vi "ASC-OvershootTest.vi"() -> ()   [LabVIEW 2009]
uses:
  <vilib>/Utility/error.llb/DialogType.ctl
  Time_globals.vi
panel:
  out "log fO2 rel. IW/IM":dbl
  out "Flush":bool
  out "Progress":string
  in  "Fugacity table":dbl[](array[numeric])
  in  "Temperature table":dbl[](array[numeric])
  out "Fugacity":cluster{"Array":dbl[], "Array 2":dbl[]}[](graph)=[{"Array"=[17.44743958824043, 17.44743958824043], "Array 2"=[-15.0, -90.0]}, {"Array"=[14.85552997103172, 14.85552997103172], "Array 2"=[-15.0, -90.0]}, {"Array"=[12.93410075664489, 12.93410075664489], "Array 2"=[-15.0, -90.0]}, {"Array"=[11.45278589016778, 11.45278589016778], "Array 2"=[-15.0, -90.0]}, {"Array"=[10.27590813338129, 10.27590813338129], "Array 2"=[-15.0, -90.0]}, {"Array"=[9.318361831989936, 9.318361831989936], "Array 2"=[-15.0, -90.0]}, {"Array"=[21.13, 21.13], "Array 2"=[-15.0, -90.0]}, {"Array"=[26.8, 26.8], "Array 2"=[-15.0, -90.0]}, {"Array"=[33.65, 33.65], "Array 2"=[-15.0, -90.0]}, {"Array"=[9.0, 11.83374083129584, 33.65, 33.65], "Array 2"=[-17.9235, -25.63552567237164, -89.48, -89.48]}, {"Array"=[], "Array 2"=[]}] caption="XY Graph"
  out "Datafile blob":string="8/29/2014\t3:28 PM\r\n\r\n0*C\r\nH2-CO2\r\nIW/IM+0\r\n\r\nTime\tSet_point\tLoad_end\tSample\tFan_end\tFan\tField\t%CO2\r\n"
  out "Start":bool
  out "Cool":bool
  out "Stable":bool
  in  "stop":bool
  out "Current SP":dbl=50.0
  out "Array":dbl[](array[numeric])
  out "refnum out":refnum<file>
  out "Fan on":bool
  in  "FAN":bool caption="Fan"
  in  "error in":errorcluster
  out "Set Point (*C)":u32
  out "Elapsed Time":dbl format="%#.0f"
  out "fan end":u32
  out "load end":u32
  out "sample":u32
  out "Watlow Chart":T1(graph)={"Number"=133, "Number"=270, "Number"=56}
  # "Temperature"
  # "Current\nTemperature"
  # "800"
  # "700"
  # "600"
  # "500"
  # "400"
  # "300"
  # "200"
  # "100"
  # "20"
  # "Temperature (*C)"
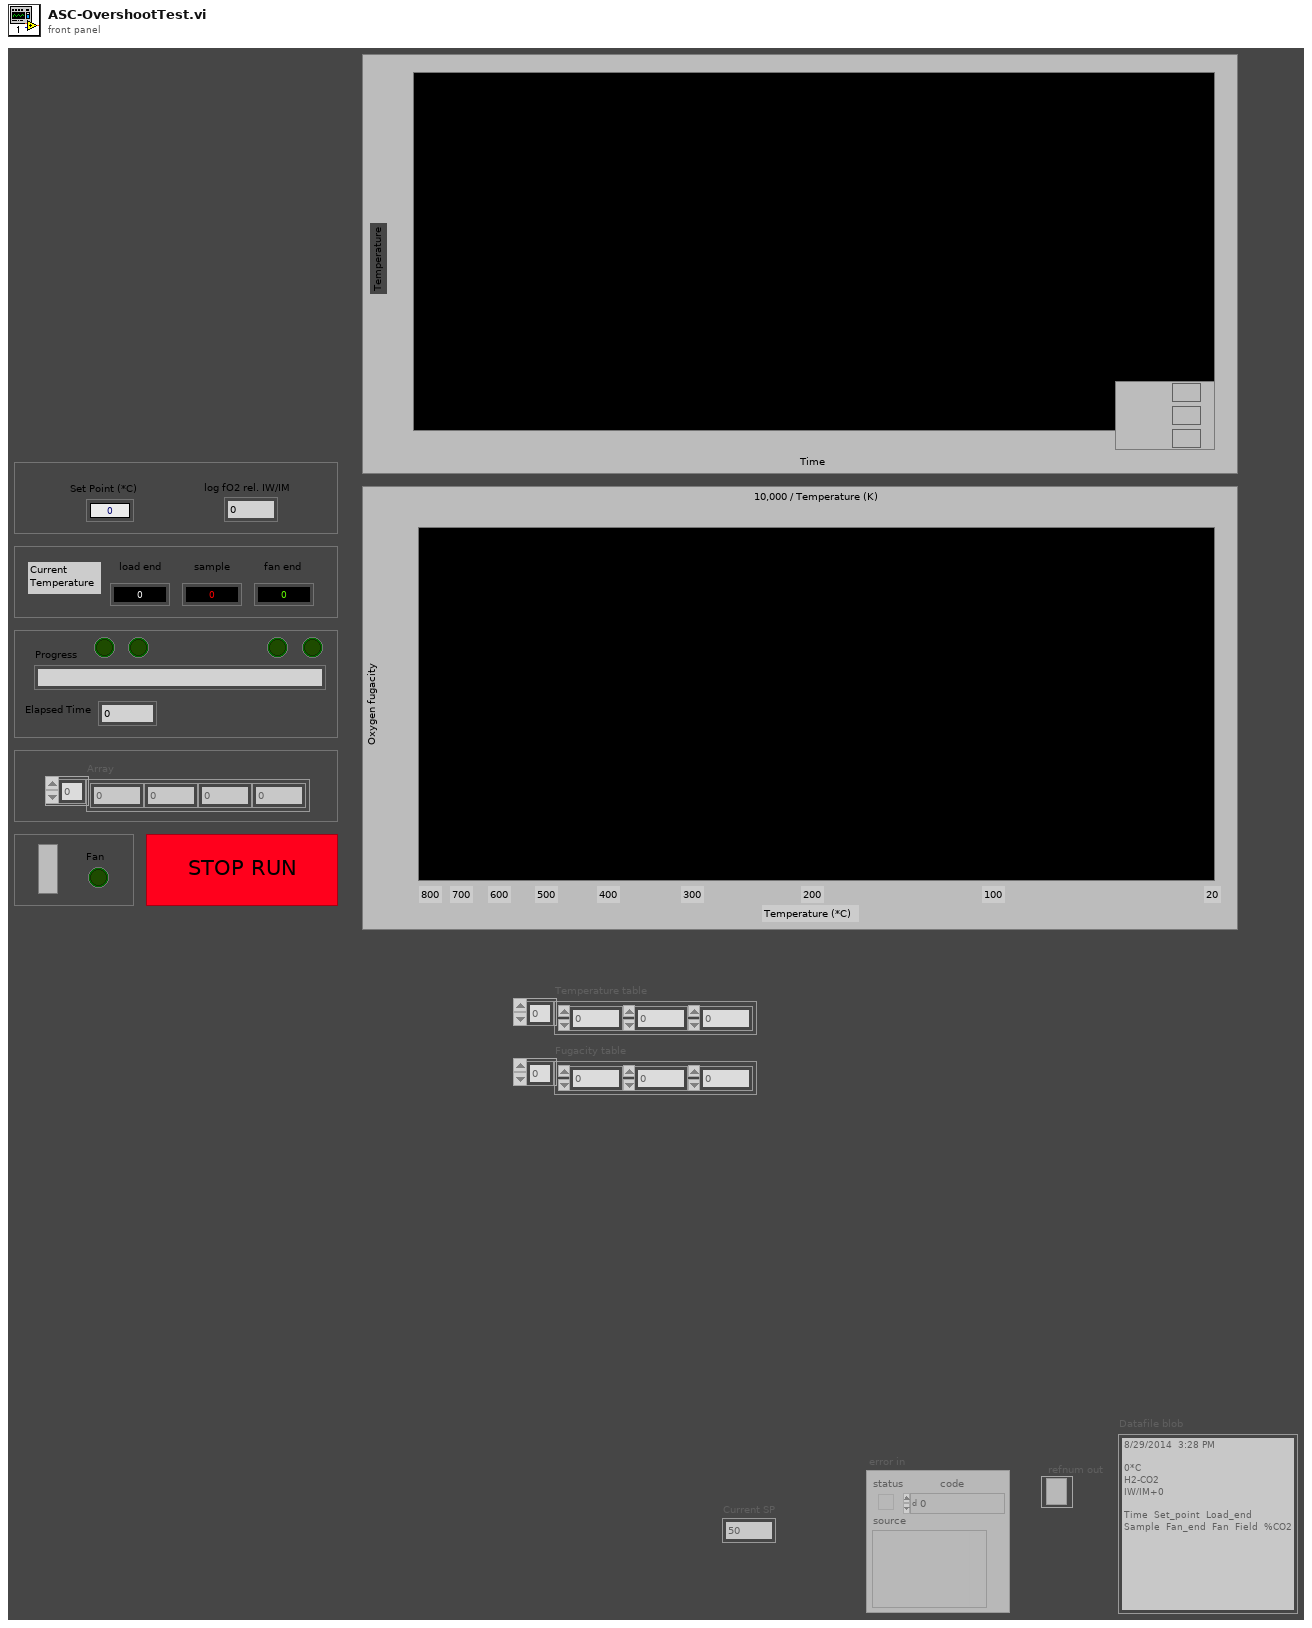
[diagram p1: front panel]
types:
  T1 = cluster{"Number":u32, "Number":u32, "Number":u32}
  T2 = cluster{"Number":u32, "Number":u32, "Number":u32}[]
  T3 = cluster{"Flow Controllers":refnum<visa-resource-name>, "Oven Fan":refnum<visa-resource-name>, "Oven Watlows":refnum<visa-resource-name>, "Field Power Supply":refnum<visa-resource-name>}
  T4 = typedef "DialogType.ctl" = u16
  T5 = cluster{"Oven Watlows":refnum<visa-resource-name>, "Field Power Supply":refnum<visa-resource-name>, "Oven Fan":refnum<visa-resource-name>, "Flow Controllers":refnum<visa-resource-name>}
  T6 = cluster{"Set Point (*C)":u32, "Number":u32, "refnum out":refnum<file>}
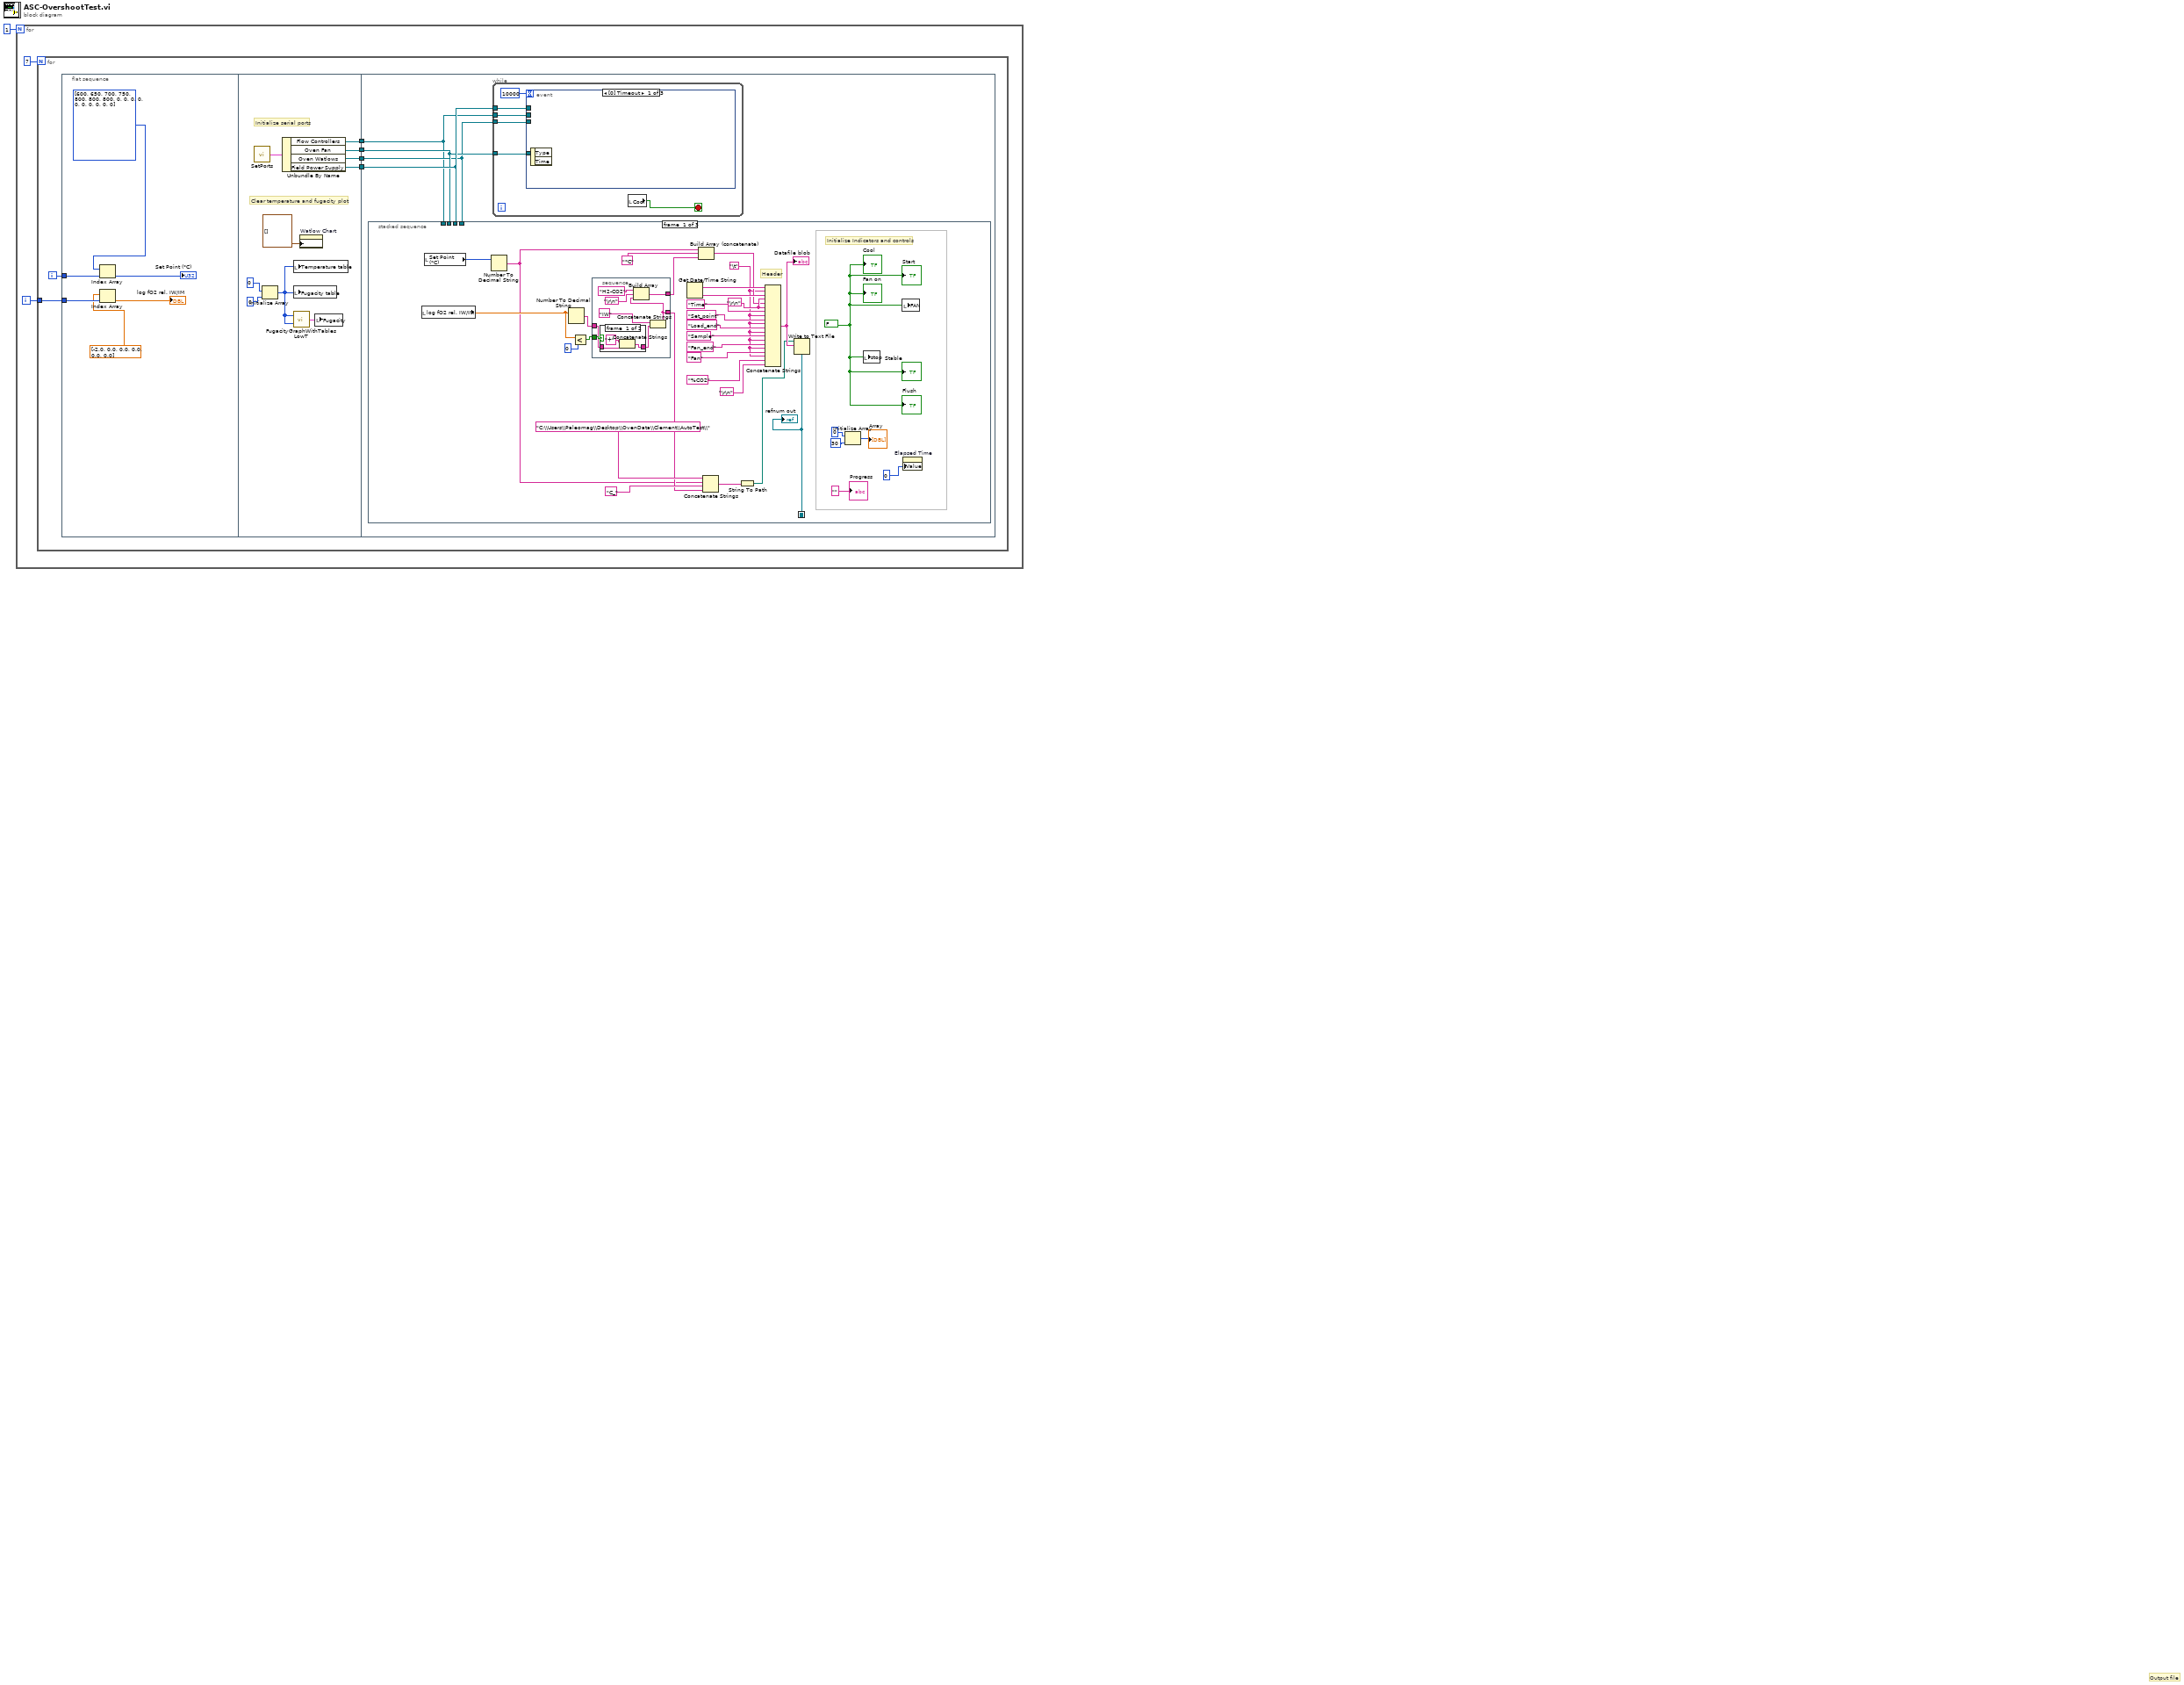
[diagram p0: block diagram]
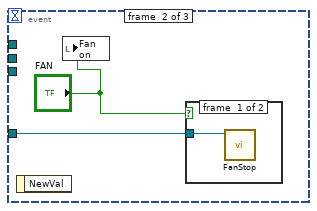
[diagram p2: hidden frame]
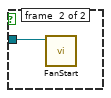
[diagram p3: hidden frame]
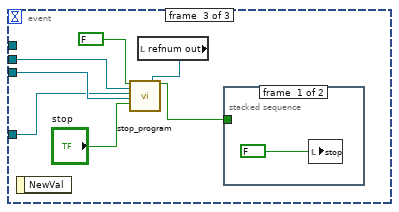
[diagram p4: hidden frame]
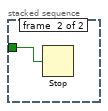
[diagram p5: hidden frame]
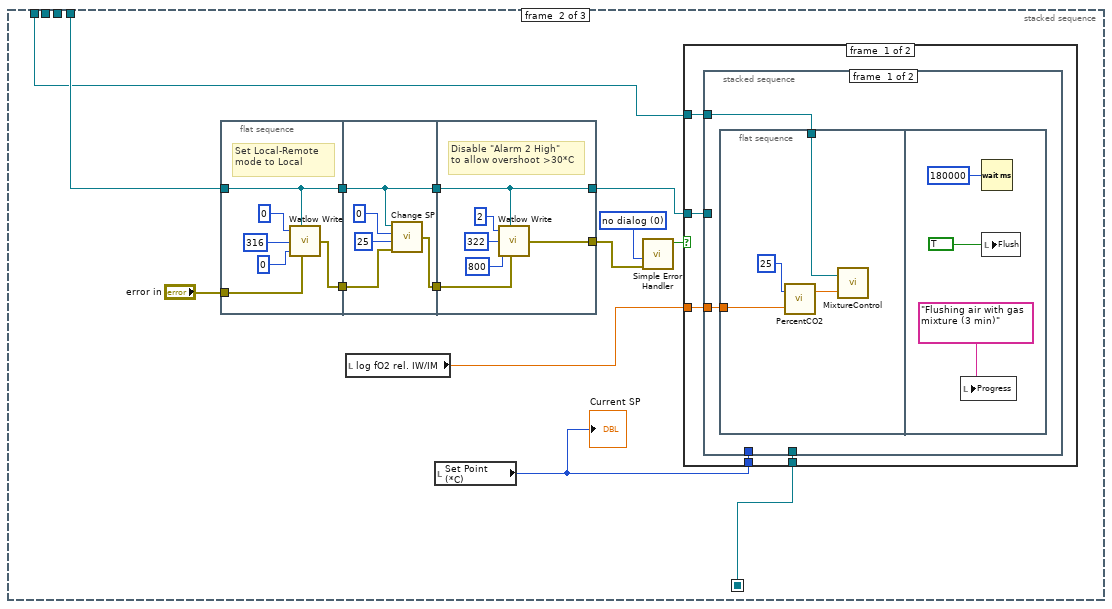
[diagram p7: hidden frame]
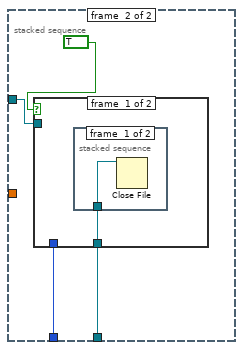
[diagram p8: hidden frame]
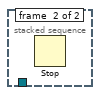
[diagram p9: hidden frame]
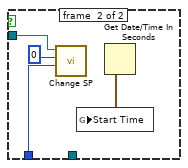
[diagram p10: hidden frame]
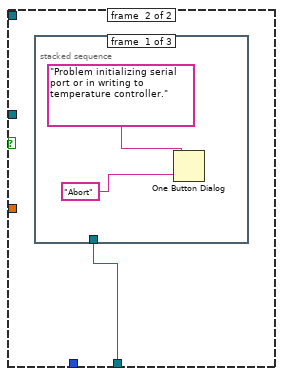
[diagram p11: hidden frame]
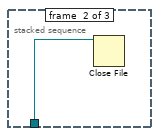
[diagram p12: hidden frame]
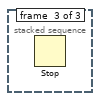
[diagram p13: hidden frame]
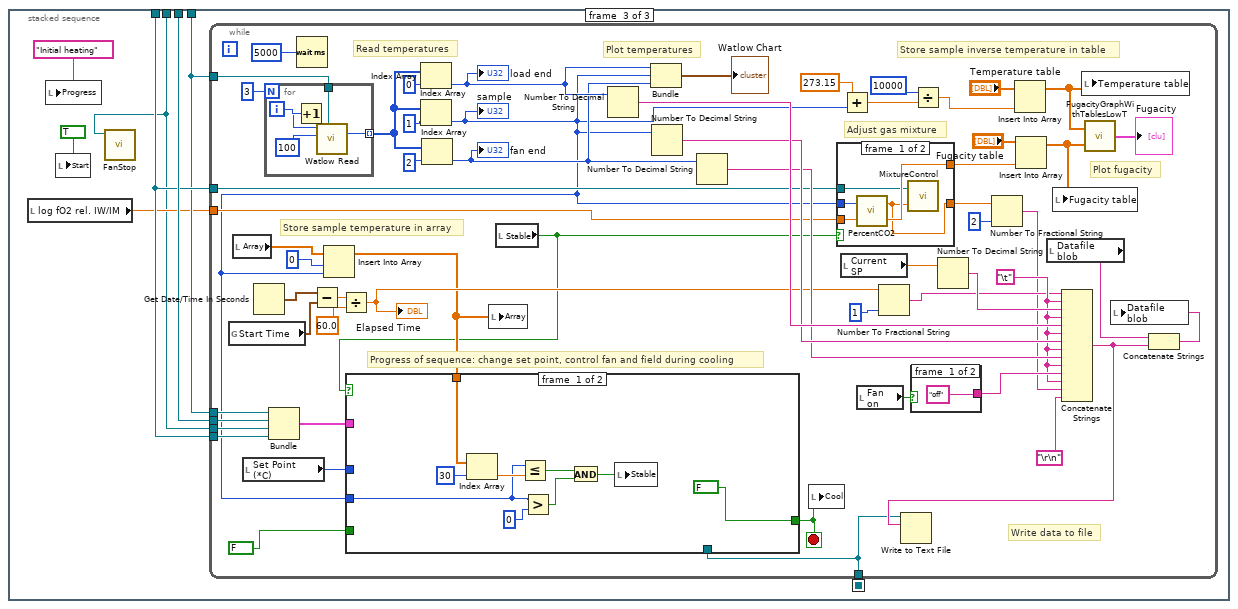
[diagram p14: hidden frame]
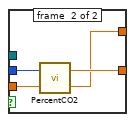
[diagram p15: hidden frame]
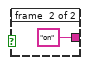
[diagram p16: hidden frame]
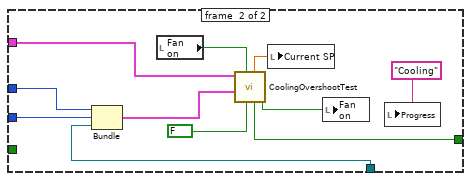
[diagram p17: hidden frame]
diagram:
  # "Output file"
  n1 = for {
    N: 1 -> [_]
    i -> [w3]
    n2 = for {
      N: 7 -> [_]
      tunnel: w3 -> [w4]
      i -> [w5]
      n3 = flat-sequence {
        tunnel: w5 -> [w15]
        tunnel: w4 -> [w14]
        tunnel: [w24] -> w9
        tunnel: [w23] -> w8
        tunnel: [w22] -> w7
        tunnel: [w19] -> w6
        tunnel: w9 -> [w29]
        tunnel: w8 -> [w28]
        tunnel: w7 -> [w27]
        tunnel: w6 -> [w26]
        frame #0 {
          n4 = Index Array(array=i32[] [600, 650, 700, 750, 800, 800, 800, 0, 0, 0, 0, 0, 0, 0, 0, 0, 0], index=w15) -> (element=→"Set Point (*C)":i32)
          n5 = Index Array(array=dbl[] [-2.0, 0.0, 0.0, 0.0, 0.0, 0.0], index=w14) -> (element=→"log fO2 rel. IW/IM":dbl)
        }
        frame #1 {
          # "Clear temperature and fugacity plot"
          # "Initialize serial ports"
          n6 = call "SetPorts.vi"() -> ("Ports"=w25:T3)  [unwired: 1 in]
          n7 = Initialize Array(0, 0) -> (w18:i32[])
          n8 = Unbundle By Name(w25) -> ("Flow Controllers"=w19:refnum<visa-resource-name>, "Oven Fan"=w23:refnum<visa-resource-name>, "Oven Watlows"=w22:refnum<visa-resource-name>, "Field Power Supply"=w24:refnum<visa-resource-name>)
          n9 = local write "Temperature table"(w18) -> ()
          n10 = local write "Fugacity table"(w18) -> ()
          n11 = call "FugacityGraphWithTablesLowT.vi"("Fugacity table"=w18, "Temperature table"=w18) -> ("Array"=w17:cluster{"Array":dbl[], "Array 2":dbl[]}[])
          n12 = property on="Watlow Chart" class="WaveformChart (strict)"("History Data"=T2 []) -> ()  [unwired: 2 in, 2 out]
          n13 = local write "Fugacity"(w17) -> ()
        }
        frame #2 {
          n14 = stacked-sequence {
            seq-local: [w58 _ _] -> [_ w98 w161]
            tunnel: w27 -> [_ w105 w156]
            tunnel: w28 -> [_ _ w154]
            tunnel: w29 -> [_ _ w159]
            tunnel: w26 -> [_ w97 w157]
            frame #0 {
              w74 = "\r\n" ("End of Line Constant")
              w61 = "\t" ("Tab Constant")
              w57 = FALSE
              # "Header"
              # "Initialize Indicators and controls"
              n15 = local read "log fO2 rel. IW/IM"() -> (w51:dbl)
              n16 = local read "Set Point (*C)"() -> (w50:u32)
              n17 = Number To Decimal String(number=w50) -> (decimal integer string=w49:string)  [unwired: 1 out]
              n18 = Number To Decimal String(number=w51) -> (decimal integer string=w65:string)  [unwired: 1 out]
              n19 = Less?(x=w51, y=0) -> (x < y?=w63:bool)
              n20 = stacked-sequence {
                tunnel: [w89] -> w70
                tunnel: w65 -> [w85]
                tunnel: w63 -> [w86]
                tunnel: [w83] -> w52
                frame #0 {
                  n21 = case shown="True" w86 {
                    tunnel: w85 -> [w92 w94]
                    tunnel: [w91 w94] -> w84
                    frame #0 {
                      n22 = Concatenate Strings("+", w92) -> (w91:string)
                    }
                    frame #1 {
                    }
                  }
                  n23 = Concatenate Strings("IW", w84) -> (w83:string)
                  n24 = Build Array("H2-CO2", "\r\n" ("End of Line Constant"), w83) -> (w89:string[])
                }
              }
              n25 = Get Date/Time String() -> (date string=w76:string, time string=w75:string)  [unwired: 3 out]
              n26 = Build Array (concatenate)(w49, "*C", w70) -> (w69:string[])
              n27 = Concatenate Strings("C:\\Users\\Paleomag\\Desktop\\OvenData\\Clement\\AutoTest\\", w49, "C_", w52) -> (w56:string)
              n28 = String To Path(string=w56) -> (path=w54:path)
              n29 = Concatenate Strings(w76, w61, w75, w74, w69, w74, "Time", w61, "Set_point", w61, "Load_end", w61, "Sample", w61, "Fan_end", w61, "Fan", w61, "%CO2", "\r\n") -> (w62:string)
              "Datafile blob" <- w62
              n30 = Write to Text File(file (use dialog)=w54, text=w62) -> (refnum out=w58:refnum<file>)  [unwired: 1 in, 3 out]
              "refnum out" <- w58
              n31 = Initialize Array(0, 30) -> (→"Array":i32[])
              n32 = local write "stop"(w57) -> ()
              n33 = local write "FAN"(w57) -> ()
              n34 = property on="Elapsed Time" class="DigNum (strict)"("Value"=0) -> ()  [unwired: 2 in, 2 out]
              "Fan on" <- w57
              "Cool" <- w57
              "Stable" <- w57
              "Start" <- w57
              "Flush" <- w57
              "Progress" <- ""
            }
            frame #1 {
              w108 = T4 0 items=["no dialog", "OK message", "continue or stop message", "OK message + warnings", "continue/stop + warnings"] ("type of dialog (OK msg:1)")
              n35 = flat-sequence {
                tunnel: w105 -> [w111]
                tunnel: [w111] -> w103
                tunnel: "error in" -> [w110]
                tunnel: [w109] -> w101
                tunnel: w103 -> [w119]
                tunnel: [w119] -> w102
                tunnel: w101 -> [w116]
                tunnel: [w115] -> w100
                tunnel: w102 -> [w120]
                tunnel: w100 -> [w125]
                tunnel: [w121] -> w99
                tunnel: [w120] -> w104
                frame #0 {
                  # "Set Local-Remote\nmode to Local"
                  n36 = call "Watlow Write.vi"("Adress"=0, "VISA resource name"=w111, "Register"=316, "Parameter"=0, "error in (no error)"=w110) -> ("error out"=w109:errorcluster)
                }
                frame #1 {
                  n37 = call "Change SP.vi"("error in"=w116, "Set Point"=25, "Adress"=0, "VISA resource name"=w119) -> ("error out"=w115:errorcluster)
                }
                frame #2 {
                  # "Disable \"Alarm 2 High\"\nto allow overshoot >30*C"
                  n38 = call "Watlow Write.vi"("Adress"=2, "VISA resource name"=w120, "Register"=322, "Parameter"=800, "error in (no error)"=w125) -> ("error out"=w121:errorcluster)
                }
              }
              n39 = local read "log fO2 rel. IW/IM"() -> (w96:dbl)
              n40 = local read "Set Point (*C)"() -> (w95:u32)
              "Current SP" <- w95
              n41 = call <vilib>:"Simple Error Handler.vi"("type of dialog (OK msg:1)"=w108, "error in (no error)"=w99) -> ("error?"=w107:bool)  [unwired: 7 out]
              n42 = case shown="False" w107 {
                tunnel: w98 -> [w130 w150]
                tunnel: w104 -> [w129 _]
                tunnel: w95 -> [w128 _]
                tunnel: w96 -> [w127 _]
                tunnel: w97 -> [w126 _]
                frame #0 {
                  n43 = stacked-sequence {
                    tunnel: w130 -> [_ w143]
                    tunnel: w129 -> [_ w142]
                    tunnel: w128 -> [_ w141]
                    tunnel: w127 -> [w131 _]
                    tunnel: w126 -> [w132 _]
                    frame #0 {
                      n44 = flat-sequence {
                        tunnel: w132 -> [w136]
                        tunnel: w131 -> [w133]
                        frame #0 {
                          n45 = call "PercentCO2.vi"("log fO2 rel. IW/IM"=w133, "Temperature"=25) -> ("%CO2"=w135:dbl)  [unwired: 1 out]
                          n46 = call "MixtureControl.vi"("%CO2"=w135, "VISA resource name"=w136) -> ()  [unwired: 1 in]
                        }
                        frame #1 {
                          n47 = local write "Progress"("Flushing air with gas mixture (3 min)") -> ()
                          n48 = Wait (ms)(milliseconds to wait=180000) -> ()  [unwired: 1 out]
                          n49 = local write "Flush"(TRUE) -> ()
                        }
                      }
                    }
                    frame #1 {
                      n50 = case shown="True" TRUE {
                        tunnel: w143 -> [w144 _]
                        tunnel: w142 -> [_ w148]
                        tunnel: w141 -> [_ w147]
                        frame #0 {
                          n51 = stacked-sequence {
                            tunnel: w144 -> [w145 _]
                            frame #0 {
                              n52 = Close File(refnum=w145) -> ()  [unwired: 1 in, 2 out]
                            }
                            frame #1 {
                              n53 = Stop() -> ()  [unwired: 1 out]
                            }
                          }
                        }
                        frame #1 {
                          n54 = call "Change SP.vi"("Set Point"=w147, "Adress"=0, "VISA resource name"=w148) -> ()  [unwired: 1 in, 1 out]
                          n55 = Get Date/Time In Seconds() -> (seconds since 1Jan1904=w149:timestamp)
                          n56 = global write "Time_globals.vi" "Start Time"(w149) -> ()
                        }
                      }
                    }
                  }
                }
                frame #1 {
                  n57 = stacked-sequence {
                    tunnel: w150 -> [_ w153 _]
                    frame #0 {
                      n58 = One Button Dialog(message="Problem initializing serial port or in writing to temperature controller.", button name ("OK")="Abort") -> ()  [unwired: 1 out]
                    }
                    frame #1 {
                      n59 = Close File(refnum=w153) -> ()  [unwired: 1 in, 2 out]
                    }
                    frame #2 {
                      n60 = Stop() -> ()  [unwired: 1 out]
                    }
                  }
                }
              }
            }
            frame #2 {
              n61 = local read "log fO2 rel. IW/IM"() -> (w155:dbl)
              n62 = local write "Progress"("Initial heating") -> ()
              n63 = local write "Start"(TRUE) -> ()
              n64 = call "FanStop.vi"("VISA resource name"=w154) -> ()  [unwired: 11 in]
              n65 = while {
                tunnel: w161 -> [w198]
                tunnel: w156 -> [w181]
                tunnel: w159 -> [w174]
                tunnel: w154 -> [w173]
                tunnel: w155 -> [w192]
                tunnel: w157 -> [w172]
                tunnel: w157 -> [w176]
                tunnel: w156 -> [w175]
                stop <- w180 stop-if-true
                w182 = "\t"
                # "Store sample temperature in array"
                # "Write data to file"
                # "Progress of sequence: change set point, control fan and field during cooling"
                # "Adjust gas mixture"
                # "Plot fugacity"
                # "Store sample inverse temperature in table"
                # "Plot temperatures"
                # "Read temperatures"
                n66 = global read "Time_globals.vi" "Start Time"() -> (w206:timestamp)
                n67 = local read "Array"() -> (w179:dbl[])
                n68 = local read "Set Point (*C)"() -> (w164:u32)
                n69 = Get Date/Time In Seconds() -> (seconds since 1Jan1904=w205:timestamp)
                n70 = for {
                  N: 3 -> [_]
                  tunnel: [w253] -> w214 mode=indexing
                  tunnel: w181 -> [w252]
                  i -> [w255]
                  n71 = Increment(x=w255) -> (x+1=w254:i32)
                  n72 = call "Watlow Read.vi"("Adress"=w254, "Register"=u8 100 ("ST-H"), "VISA resource name"=w252) -> ("Number"=w253:u32)  [unwired: 1 in, 2 out]
                }
                n73 = Bundle("Oven Watlows"=w175, "Field Power Supply"=w174, "Oven Fan"=w173, "Flow Controllers"=w172) -> (w171:T5)  [unwired: 1 in]
                n74 = Wait (ms)(milliseconds to wait=u32 5000) -> ()  [unwired: 1 out]
                n75 = Subtract(x=w205, y=w206) -> (x-y=w207:dbl)
                n76 = Divide(x=w207, y=60.0) -> (x/y=w204:dbl)
                "Elapsed Time" <- w204
                n77 = Index Array(array=w214, index=0) -> (element=w210:u32)
                "load end" <- w210
                n78 = Index Array(array=w214, index=1) -> (element=w167:u32)
                "sample" <- w167
                n79 = Insert Into Array(array=w179, index=0, new element=w167) -> (w163:dbl[])
                n80 = Index Array(array=w214, index=2) -> (element=w209:u32)
                "fan end" <- w209
                n81 = local write "Array"(w163) -> ()
                n82 = local read "Stable"() -> (w162:bool)
                n83 = case shown="False" w162 {
                  tunnel: w198 -> [_ w243]
                  tunnel: [FALSE w247] -> w180
                  tunnel: w164 -> [_ w249]
                  tunnel: w167 -> [w235 w248]
                  tunnel: FALSE -> [_ _]
                  tunnel: w163 -> [w237 _]
                  tunnel: w171 -> [_ w242]
                  frame #0 {
                    n84 = Index Array(array=w237, index=30) -> (element=w238:dbl)
                    n85 = Less Or Equal?(x=w235, y=w238) -> (x <= y?=w232:bool)
                    n86 = Greater?(x=w235, y=0) -> (0:w233:bool)
                    n87 = And(x=w232, y=w233) -> (x .and. y?=w231:bool)
                    n88 = local write "Stable"(w231) -> ()
                  }
                  frame #1 {
                    n89 = Bundle("Set Point (*C)"=w249, "Number"=w248, "refnum out"=w243) -> (w240:T6)  [unwired: 1 in]
                    n90 = local read "Fan on"() -> (w246:bool)
                    n91 = call "CoolingOvershootTest.vi"("Read Field"=FALSE, "Read Fan"=w246, "Cluster"=w240, "Ports"=w242) -> ("Fan on"=w245:bool, "Run complete"=w247:bool, "Current SP"=w244:dbl)  [unwired: 4 in, 1 out]
                    n92 = local write "Current SP"(w244) -> ()
                    n93 = local write "Fan on"(w245) -> ()
                    n94 = local write "Progress"("Cooling") -> ()
                  }
                }
                n95 = Number To Decimal String(number=w210) -> (decimal integer string=w219:string)  [unwired: 1 out]
                n96 = Bundle("Number"=w210, "Number"=w167, "Number"=w209) -> (→"Watlow Chart":T1)  [unwired: 1 out]
                n97 = Number To Decimal String(number=w167) -> (decimal integer string=w213:string)  [unwired: 1 out]
                n98 = Number To Decimal String(number=w209) -> (decimal integer string=w212:string)  [unwired: 1 out]
                n99 = local write "Cool"(w180) -> ()
                n100 = case shown="False" w162 {
                  tunnel: w192 -> [w224 w227]
                  tunnel: w167 -> [w223 w228]
                  tunnel: [w222 w225] -> w185
                  tunnel: [w221 w226] -> w178
                  tunnel: w176 -> [w220 _]
                  frame #0 {
                    n101 = call "PercentCO2.vi"("log fO2 rel. IW/IM"=w224, "Temperature"=w223) -> ("Fugacity"=w222:dbl, "%CO2"=w221:dbl)
                    n102 = call "MixtureControl.vi"("%CO2"=w221, "VISA resource name"=w220) -> ()  [unwired: 1 in]
                  }
                  frame #1 {
                    n103 = call "PercentCO2.vi"("log fO2 rel. IW/IM"=w227, "Temperature"=w228) -> ("Fugacity"=w225:dbl, "%CO2"=w226:dbl)
                  }
                }
                n104 = local read "Current SP"() -> (w177:dbl)
                n105 = Add(x=273.15, y=w167) -> (x+y=w189:dbl)
                n106 = local read "Fan on"() -> (w196:bool)
                n107 = Number To Fractional String(number=w204, precision (6)=i16 1) -> (F-format string=w170:string)  [unwired: 2 out]
                n108 = case shown="True" w196 {
                  tunnel: ["off" "on"] -> w200
                  frame #0 {
                  }
                  frame #1 {
                  }
                }
                n109 = Divide(x=10000, y=w189) -> (x/y=w187:dbl)
                n110 = Number To Decimal String(number=w177) -> (decimal integer string=w201:string)  [unwired: 1 out]
                n111 = Number To Fractional String(number=w178, precision (6)=2) -> (F-format string=w168:string)  [unwired: 2 in]
                n112 = Insert Into Array(array="Temperature table", new element=w187) -> (w186:dbl[])  [unwired: 1 in]
                n113 = Insert Into Array(array="Fugacity table", new element=w185) -> (w184:dbl[])  [unwired: 1 in]
                n114 = local read "Datafile blob"() -> (w195:string)
                n115 = local write "Fugacity table"(w184) -> ()
                n116 = Concatenate Strings(w170, w182, w201, w182, w219, w182, w213, w182, w212, w182, w200, w182, w168, "\r\n") -> (w202:string)
                n117 = Write to Text File(file (use dialog)=w198, text=w202) -> ()  [unwired: 1 in, 4 out]
                n118 = local write "Temperature table"(w186) -> ()
                n119 = call "FugacityGraphWithTablesLowT.vi"("Fugacity table"=w184, "Temperature table"=w186) -> ("Array"=→"Fugacity":cluster{"Array":dbl[], "Array 2":dbl[]}[])
                n120 = Concatenate Strings(w195, w202) -> (w194:string)
                n121 = local write "Datafile blob"(w194) -> ()
              }
            }
          }
          n122 = while {
            tunnel: w27 -> [w35]
            tunnel: w28 -> [w34]
            tunnel: w29 -> [w33]
            tunnel: w26 -> [w32]
            stop <- w31 stop-if-true
            n123 = event shown="[0] Timeout" {
              selector: _ -> [_ _ _]
              dyn-events: _ -> [_ _ _]
              timeout: 10000 -> [_ _ _]
              tunnel: w35 -> [_ _ w43]
              tunnel: w34 -> [_ w36 w42]
              tunnel: w33 -> [_ _ _]
              tunnel: w32 -> [_ _ w41]
              event #0 {
                n124 = event-data() -> ()  [unwired: 1 in, 2 out]
              }
              event #1 {
                n125 = event-data() -> ()  [unwired: 1 in, 1 out]
                n126 = local write "Fan on"("FAN") -> ()
                n127 = case shown="True" "FAN" {
                  tunnel: w36 -> [w38 w39]
                  frame #0 {
                    n128 = call "FanStop.vi"("VISA resource name"=w38) -> ()  [unwired: 11 in]
                  }
                  frame #1 {
                    n129 = call "FanStart.vi"("VISA resource name"=w39) -> ()  [unwired: 11 in]
                  }
                }
              }
              event #2 {
                n130 = event-data() -> ()  [unwired: 1 in, 1 out]
                n131 = local read "refnum out"() -> (w40:refnum<file>)
                n132 = call "stop_program.vi"("Run complete"=FALSE, "Flow Controllers"=w41, "Fan"=w42, "Watlows"=w43, "stop"="stop", "filename"=w40) -> ("Reset?"=w46:bool)  [unwired: 12 in, 1 out]
                n133 = stacked-sequence {
                  tunnel: w46 -> [_ w48]
                  frame #0 {
                    n134 = local write "stop"(FALSE) -> ()
                  }
                  frame #1 {
                    n135 = Stop(stop? (T)=w48) -> ()
                  }
                }
              }
            }
            n136 = local read "Cool"() -> (w31:bool)
          }
        }
      }
    }
  }
